vi "Launch and Monitor Command.vi"() -> ()   [LabVIEW 2013]
uses:
  USER32.DLL
panel:
  out "error out":errorcluster
  out "Clipboard:Read From Clipboard":string
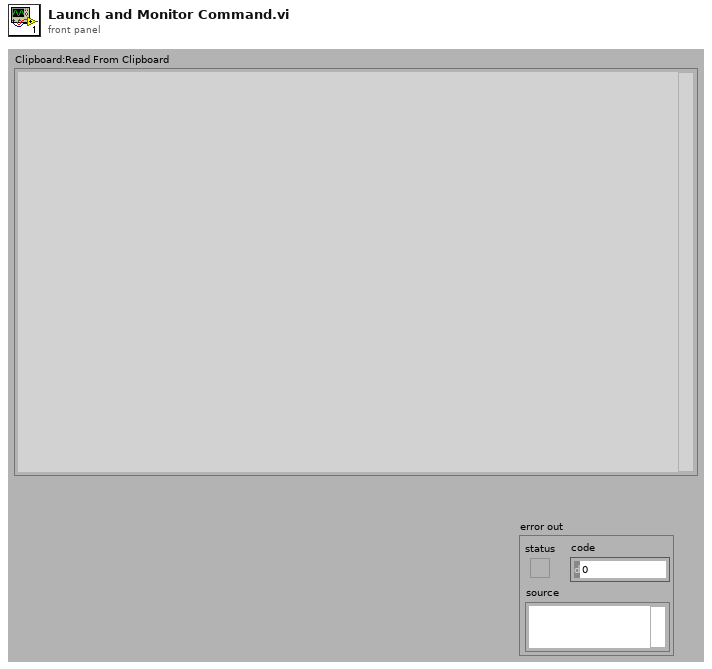
[diagram p1: front panel]
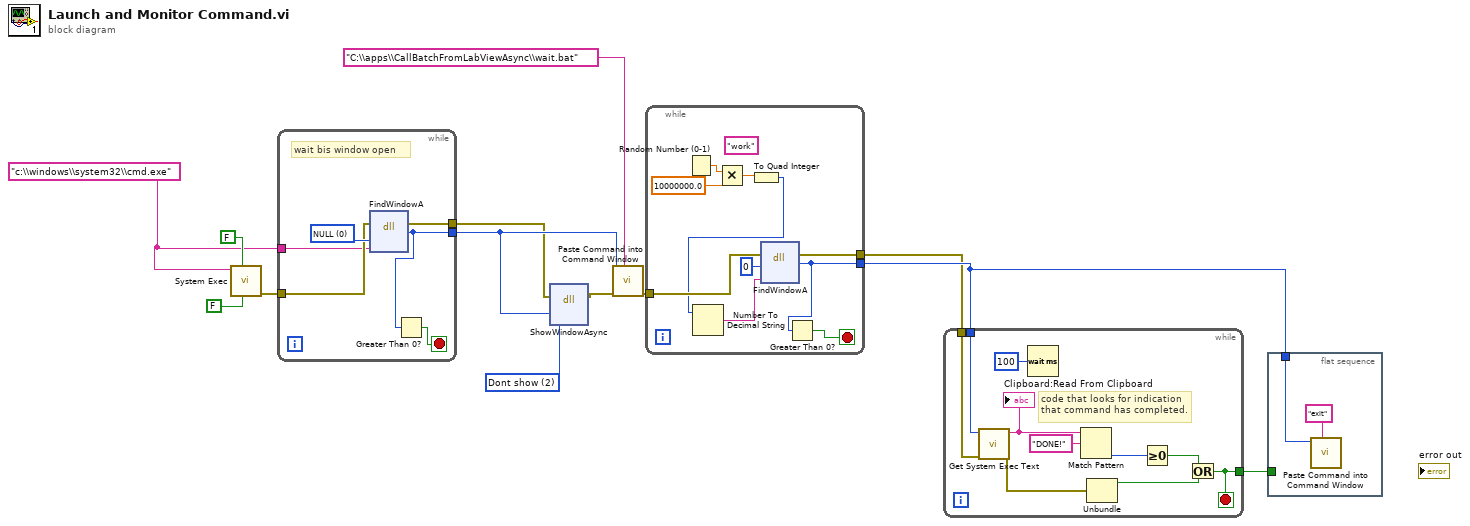
[diagram p0: block diagram]
diagram:
  w7 = u16 2 items=["Dont show"=2, "Show"=1] ("mCmdShow")
  w10 = "c:\\windows\\system32\\cmd.exe" ("command line")
  n1 = call <vilib>:"System Exec.vi"("run minimized? (F)"=FALSE, "wait until completion? (T)"=FALSE, "command line"=w10) -> ("error out"=w8:errorcluster)  [unwired: 5 in, 3 out]
  n2 = while {
    tunnel: w10 -> [w14]
    tunnel: [w15] -> w6
    tunnel: w8 -> [w18]
    tunnel: [w17] -> w5
    stop <- w16 stop-if-true
    w19 = 0 items=["NULL"]
    # "wait bis window open"
    n3 = dll-call lib="USER32.DLL" fn="FindWindowA" label="FindWindow"(error in=w18, "lpszClassName"=w19, "lpszWindowName"=w14) -> (error out=w17:errorcluster, "hWnd"=w15:u32)  [unwired: 4 in, 1 out]
    n4 = Greater Than 0?(x=w15) -> (x > 0?=w16:bool)
  }
  n5 = dll-call lib="USER32.DLL" fn="ShowWindowAsync" label="FindWindow"(error in=w5, "hWnd"=w6, "mCmdShow"=w7) -> (error out=w4:errorcluster)  [unwired: 5 in, 1 out]
  n6 = call "Paste Command into Command Window.vi"("command"="C:\\apps\\CallBatchFromLabViewAsync\\wait.bat", "error in (no error)"=w4, "hWnd"=w6) -> ("error out"=w3:errorcluster)  [unwired: 8 in]
  n7 = while {
    tunnel: w3 -> [w29]
    tunnel: [w27] -> w2
    tunnel: [w25] -> w1
    stop <- w26 stop-if-true
    (unwired) "work" ("lpszWindowName")
    n8 = Random Number (0-1)() -> (number: 0 to 1=w24:dbl)
    n9 = Multiply(x=w24, y=10000000.0) -> (x*y=w22:dbl)
    n10 = To Quad Integer(1:w22) -> (0:w21:i64)
    n11 = Number To Decimal String(number=w21) -> (decimal integer string=w20:string)  [unwired: 1 in]
    n12 = dll-call lib="USER32.DLL" fn="FindWindowA" label="FindWindow"(error in=w29, "lpszClassName"=0, "lpszWindowName"=w20) -> (error out=w25:errorcluster, "hWnd"=w27:u32)  [unwired: 4 in, 1 out]
    n13 = Greater Than 0?(x=w27) -> (x > 0?=w26:bool)
  }
  n14 = while {
    tunnel: w2 -> [w31]
    tunnel: [w32] -> w12
    tunnel: w1 -> [w30]
    stop <- w32 stop-if-true
    # "code that looks for indication that command has completed."
    n15 = call "Get System Exec Text.vi"("error in (no error)"=w30, "hWnd"=w31) -> ("error out"=w36:errorcluster, "Clipboard:Read From Clipboard"=w38:string)  [unwired: 8 in]
    "Clipboard:Read From Clipboard" <- w38
    n16 = Wait (ms)(milliseconds to wait=u32 100) -> ()  [unwired: 1 out]
    n17 = Match Pattern(string=w38, regular expression="DONE!") -> (offset past match=w34:i32)  [unwired: 1 in, 3 out]
    n18 = Unbundle(w36) -> ("status"=w35:bool)  [unwired: 2 out]
    n19 = Greater Or Equal To 0?(x=w34) -> (x >= 0?=w33:bool)
    n20 = Or(x=w33, y=w35) -> (x .or. y?=w32:bool)
  }
  n21 = flat-sequence {
    tunnel: w12 -> [_]
    tunnel: w2 -> [w41]
    frame #0 {
      n22 = call "Paste Command into Command Window.vi"("command"="exit", "hWnd"=w41) -> ()  [unwired: 9 in, 1 out]
    }
  }
